vi "SC TCP Unflatten String.vi"(8 "error in":errorcluster, 11 "Response JSON":string) -> (0 "error out":errorcluster, 1 "Command Completed":bool, 3 "Return Data":string)   [LabVIEW 2018]
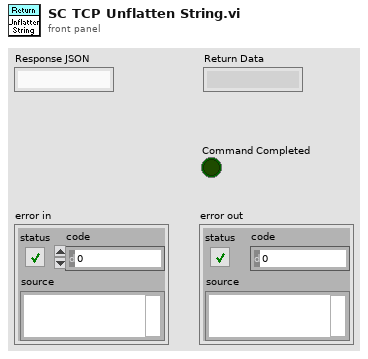
[diagram p1: front panel]
types:
  T1 = cluster{"cmdCompleted":bool, "returnData":cluster{"Value":string}}
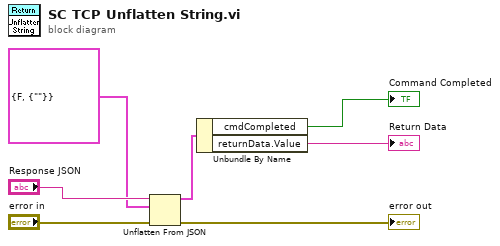
[diagram p0: block diagram]
diagram:
  n1 = Unflatten From JSON(JSON string="Response JSON", type and defaults=T1 {"cmdCompleted"=FALSE, "returnData"={"Value"=""}} ("Response Details"), error in (no error)="error in") -> (value=w3:T1, error out=→"error out":errorcluster)  [unwired: 4 in]
  n2 = Unbundle By Name(w3) -> ("cmdCompleted"=→"Command Completed":bool, "returnData.Value"=→"Return Data":string)
